vi "Transmit Data over TCP.vi"() -> ()   [LabVIEW 2023]
uses:
  Type Definitions/Payload Class.ctl
  Type Definitions/Data Frame Header.ctl
  Type Definitions/Data Frame.ctl
  Type Definitions/Telemetry TCP State.ctl
  <vilib>/Platform/TimedLoop/XDataNode/wakeup.ctl
  <vilib>/Platform/TimedLoop/XDataNode/XDNodeRunTimeDep.lvlib
  <vilib>/Platform/TimedLoop/XDataNode/nitl_modes.ctl
  <vilib>/Platform/TimedLoop/XDataNode/timing_clust.ctl
  <vilib>/platform/TimedLoop/XDataNode/XDataNode.xnode
  Type Definitions/Enum - System State.ctl
  Type Definitions/Device.ctl
panel:
  out "Is Connected":bool
  out "Remote Port":u16
  out "Frames Sent":i32
  out "Bytes Sent":i32
  out "Remote Address":string
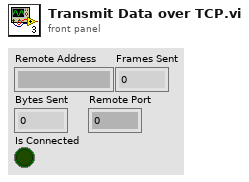
[diagram p1: front panel]
types:
  T1 = typedef "XDNodeRunTimeDep.lvlib/timing_clust.ctl" = cluster{"Expected End [f-1]":u64, "Actual End [f-1]":u64, "Finished Late? [f-1]":bool, "Expected End [i-1]":u64, "Actual End [i-1]":u64, "Finished Late? [i-1]":bool, "Expected Start [i]":u64, "Actual Start [i]":u64, "Expected Start [f]":u64, "Actual Start [f]":u64, "Source Name":string, "Structure Name":string, "Period":i64, "Deadline":i64, "Offset":i64, "Start":i64, "Priority":i32, "Timeout":i32, "Mode":T2, "Wakeup Reason":T3, "Error":errorcluster, "Source Type":string, "Secondary Source Type":string, "Global End Time":u64, "Global Start Time":u64, "Frame Duration":u64, "Iteration Duration":u64, "Assigned CPU":i32, "I/O Scan Engine Mode":u32}
  T2 = typedef "XDNodeRunTimeDep.lvlib/nitl_modes.ctl" = enum32{"No Change", "Process missed periods, maintain original phase", "Discard missed periods, maintain original phase", "Process missed periods, ignore original phase", "Discard missed periods, ignore original phase"}
  T3 = typedef "XDNodeRunTimeDep.lvlib/wakeup.ctl" = enum32{"Normal", "Aborted", "Asynchronous wakeup", "Timing source error", "Timed loop error", "Timeout"}
  T4 = typedef "Data Frame.ctl" = cluster{"Frame Header":T5, "Payload":string, "CRC":u32}
  T5 = typedef "Data Frame Header.ctl" = cluster{"Sync":u32, "Time":dbl, "Nanosecond Counter":i64, "Payload Class":T6, "Payload ID":u16, "Counter":i32, "Options":u32, "Source":T7, "Destination":T7}
  T6 = typedef "Payload Class.ctl" = enum16{"System State", "Parameters", "Metadata", "Software Monitor", "Data", "Commands"}
  T7 = typedef "Device.ctl" = enum32{"None", "Exec", "Aux1", "Aux2", "Aux3"}
  T8 = typedef "Enum - System State.ctl" = enum16{"System Time", "Telemetry TCP State", "Writeable Drive State", "Command TCP State", "Network Adapter State", "Discovery Engine State", "Disk State"}
  T9 = typedef "Telemetry TCP State.ctl" = cluster{"Is Connected":bool, "Remote Address":string, "Remote Port":u16, "Total Frames Sent":i32, "Total Bytes Sent":i32}
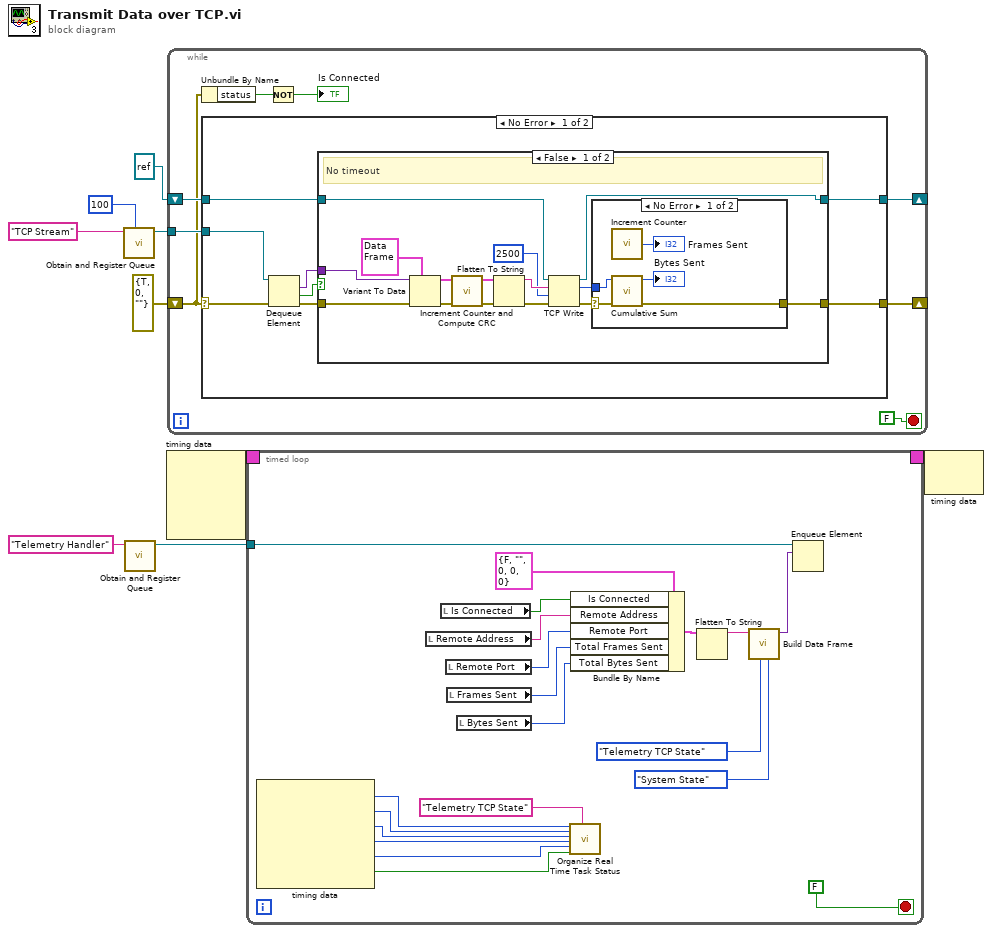
[diagram p0: block diagram]
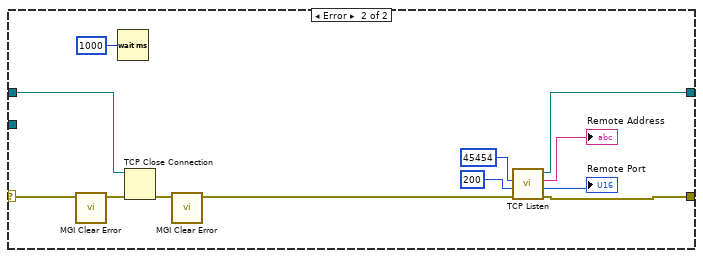
[diagram p4: hidden frame]
diagram:
  n1 = call "Obtain and Register Queue.vi"("max queue size (-1, unlimited)"=100, "Queue Name (unnamed)"="TCP Stream" ("name (unnamed)")) -> ("Queue Reference"=w6:refnum<queue>)  [unwired: 8 in, 1 out]
  n2 = call "Obtain and Register Queue.vi"("Queue Name (unnamed)"="Telemetry Handler" ("name (unnamed)")) -> ("Queue Reference"=w2:refnum<queue>)  [unwired: 9 in, 1 out]
  n3 = node-c288() -> (w4:T1)  [unwired: 4 in]
  n4 = while {
    shift-right: [w17] -> _
    shift-left: errorcluster {"status"=TRUE, "code"=0, "source"=""} ("error out") -> [w12]
    shift-right: [w13] -> _
    shift-left: refnum<k5> refnum ("connection ID") -> [w16]
    tunnel: w6 -> [w15]
    stop <- FALSE stop-if-true
    n5 = Unbundle By Name(w12) -> ("status"=w11:bool)
    n6 = case shown="No Error" w12 {
      selector: w12 -> [w24 w50]
      tunnel: [w19 w55] -> w17
      tunnel: [w20 w57] -> w13
      tunnel: w16 -> [w23 w59]
      tunnel: w15 -> [w25 _]
      frame No Error {
        n7 = Dequeue Element(queue=w25, error in (no error)=w24) -> (element=w22:variant, timed out?=w18:bool, error out=w21:errorcluster)  [unwired: 1 in, 1 out]
        n8 = case shown="False" w18 {
          tunnel: w23 -> [w40 w47]
          tunnel: w22 -> [w38 _]
          tunnel: w21 -> [w35 w48]
          tunnel: [w31 w47] -> w20
          tunnel: [w27 w48] -> w19
          frame False {
            # "No timeout"
            n9 = Variant To Data(error in=w35, type=T4 {"Frame Header"={"Sync"=0, "Time"=0.0, "Nanosecond Counter"=0, "Payload Class"=enum."System State", "Payload ID"=0, "Counter"=0, "Options"=0, "Source"=enum."None", "Destination"=enum."None"}, "Payload"="", "CRC"=0} ("Frame"), Variant=w38) -> (data=w39:T4, error out=w34:errorcluster)
            n10 = call "Increment Counter and Compute CRC.vi"("error in (no error)"=w34, "Frame In"=w39) -> ("error out"=w33:errorcluster, "Frame Out"=w29:T4)  [unwired: 8 in]
            n11 = Flatten To String(anything=w29, error in (no error)=w33) -> (data string=w36:string, error out=w32:errorcluster)  [unwired: 2 in, 1 out]
            n12 = TCP Write(connection ID=w40, data in=w36, error in (no error)=w32, 9:2500 ("timeout ms (25000)")) -> (connection ID out=w31:refnum<k5>, bytes written=w30:i32, error out=w26:errorcluster)
            n13 = case shown="No Error" w26 {
              selector: w26 -> [w42 w46]
              tunnel: w30 -> [w43 _]
              tunnel: [w41 w46] -> w27
              frame No Error {
                n14 = call "Increment Counter.vi"() -> ("Count"=→"Frames Sent":i32)  [unwired: 5 in]
                n15 = call "Cumulative Sum.vi"("error in (no error)"=w42, "Value In"=w43) -> ("error out"=w41:errorcluster, "Cumulative Sum"=→"Bytes Sent":i32)  [unwired: 8 in]
              }
              frame Error {
              }
            }
          }
          frame True {
            # "Timed out"
          }
        }
      }
      frame Error {
        n16 = call <userlib>:"MGI Clear Error.vi"("Error In"=w50) -> ("Error Out"=w49:errorcluster)  [unwired: 6 in]
        n17 = Wait (ms)(milliseconds to wait=u32 1000) -> ()  [unwired: 1 out]
        n18 = TCP Close Connection(connection ID=w59, error in (no error)=w49) -> (error out=w58:errorcluster)  [unwired: 1 in, 1 out]
        n19 = call <userlib>:"MGI Clear Error.vi"("Error In"=w58) -> ("Error Out"=w56:errorcluster)  [unwired: 6 in]
        n20 = call <vilib>:"TCP Listen.vi"("error in (no error)"=w56, "timeout ms (wait forever: -1)"=200, "port"=u16 45454) -> ("error out"=w55:errorcluster, "remote port"=→"Remote Port":u16, "remote address"=→"Remote Address":string, "connection ID"=w57:refnum<k5>)  [unwired: 4 in, 1 out]
      }
    }
    n21 = Not(x=w11) -> (.not. x?=→"Is Connected":bool)
  }
  n22 = timed-loop {
    timing: w4 -> [_]
    timing-out: [_] -> w3
    tunnel: w2 -> [w68]
    stop <- FALSE stop-if-true
    n23 = node-c288() -> (w78:i32, w77:i32, w76:i64, w75:i64, w74:i64, w73:bool)  [unwired: 1 in]
    n24 = local read "Remote Address"() -> (w65:string)
    n25 = local read "Is Connected"() -> (w61:bool)
    n26 = local read "Remote Port"() -> (w64:u16)
    n27 = local read "Frames Sent"() -> (w63:i32)
    n28 = local read "Bytes Sent"() -> (w62:i32)
    n29 = call "Organize Real Time Task Status.vi"("Priority"=w78, "Processor"=w77, "Offset"=w76, "Iteration Duration"=w75, "Period"=w74, "Finished Late? [i-1]"=w73, "Task Name"="Telemetry TCP State") -> ()  [unwired: 12 in, 1 out]
    n30 = Bundle By Name(cluster=T9 {"Is Connected"=FALSE, "Remote Address"="", "Remote Port"=0, "Total Frames Sent"=0, "Total Bytes Sent"=0} ("Cluster"), "Is Connected"=w61, "Remote Address"=w65, "Remote Port"=w64, "Total Frames Sent"=w63, "Total Bytes Sent"=w62) -> (w67:T9)
    n31 = Flatten To String(anything=w67) -> (data string=w70:string)  [unwired: 3 in, 2 out]
    n32 = call "Build Data Frame.vi"("Payload Class (Data)"=Payload_Class."System State", "Payload ID (0)"=Enum_-_System_State."Telemetry TCP State" ("System State"), "Payload (Empty String)"=w70) -> ("Frame"=w69:variant)  [unwired: 7 in, 1 out]
    n33 = Enqueue Element(queue=w68, element=w69) -> ()  [unwired: 2 in, 3 out]
  }
  n34 = node-c288(w3) -> ()  [unwired: 1 out]
